vi "configure operation.vi"(7 "tag bus configurable plugin module configuration":refnum<class "Modbus Slave configuration.lvclass">, 8 "error in":errorcluster, 10 "line item in":T2, 11 "engine configuration":refnum<class "engine configuration.lvclass">) -> (0 "error out":errorcluster, 1 "success":bool, 2 "line item out":T2, 5 "changed":bool)   [LabVIEW 2013, in "Modbus Slave editor node.lvclass"]
doc: "Platypus Framework 1.0.1.65\nNI Systems Engineering - National Instruments"
uses:
  Modbus Slave editor node.lvclass
  permissions.ctl
  table line.ctl
  <vilib>/NI/TBM Modules/modbus slave/module channel/Modbus Module Channel.lvclass
  <vilib>/NI/Module Execution Interface/Engine Configuration/engine configuration.lvclass
  <vilib>/NI/TBM Modules/modbus slave/configuration/Modbus Slave configuration.lvclass
  <vilib>/NI/TBM Modules/modbus slave/module channel/data bank type.ctl
  <vilib>/NI/Tag Bus Module Framework/root configuration/TBM configuration.lvclass/TBM configuration.ctl
  <vilib>/NI/Tag Bus Module Framework/channel/TBM channel.lvclass/TBM channel.ctl
  <vilib>/NI/TBM Modules/modbus slave/module channel/Modbus Module Channel.lvclass/Modbus Module Channel.ctl
  <vilib>/NI/Tag Bus/tag/tag descriptor.lvclass/tag descriptor.ctl
  <vilib>/NI/Tag Bus/tag/Data Type.ctl
  <vilib>/NI/Tag Bus Module Framework/channel/Read channel classification.vi
  <vilib>/NI/TBM Modules/modbus slave/module channel/Read modbus type.vi
  <vilib>/NI/TBM Modules/modbus slave/module channel/Read starting address.vi
  <vilib>/NI/TBM Modules/modbus slave/module channel/Read subindex (bool).vi
  <vilib>/NI/Tag Bus/tag/read data type.vi
  <vilib>/NI/Tag Bus Module Framework/root configuration/Read instance name.vi
  <vilib>/NI/Tag Bus/tag/write data type.vi
  <vilib>/NI/Tag Bus Module Framework/channel/Write channel classification.vi
  <vilib>/NI/TBM Modules/modbus slave/module channel/Write modbus type.vi
  <vilib>/NI/TBM Modules/modbus slave/module channel/Write starting address.vi
  <vilib>/NI/TBM Modules/modbus slave/module channel/Write subindex (bool).vi
  <vilib>/NI/Tag Bus/tag/write tag name.vi
  <vilib>/NI/Tag Bus Module Framework/root configuration/create GUID.vi
  <vilib>/NI/Tag Bus/tag/tag descriptor.lvclass
panel:
  out "issues":string
  in  "Tag":i32(listbox)
  in  "Type":i32(listbox)
  in  "Bit":i32 min=0 max=15 step=1
  in  "Address (0 index)":i32
  in  "modbus bank":T1
  in  "cancel":bool
  in  "ok":bool
  in  "Access Type":T3
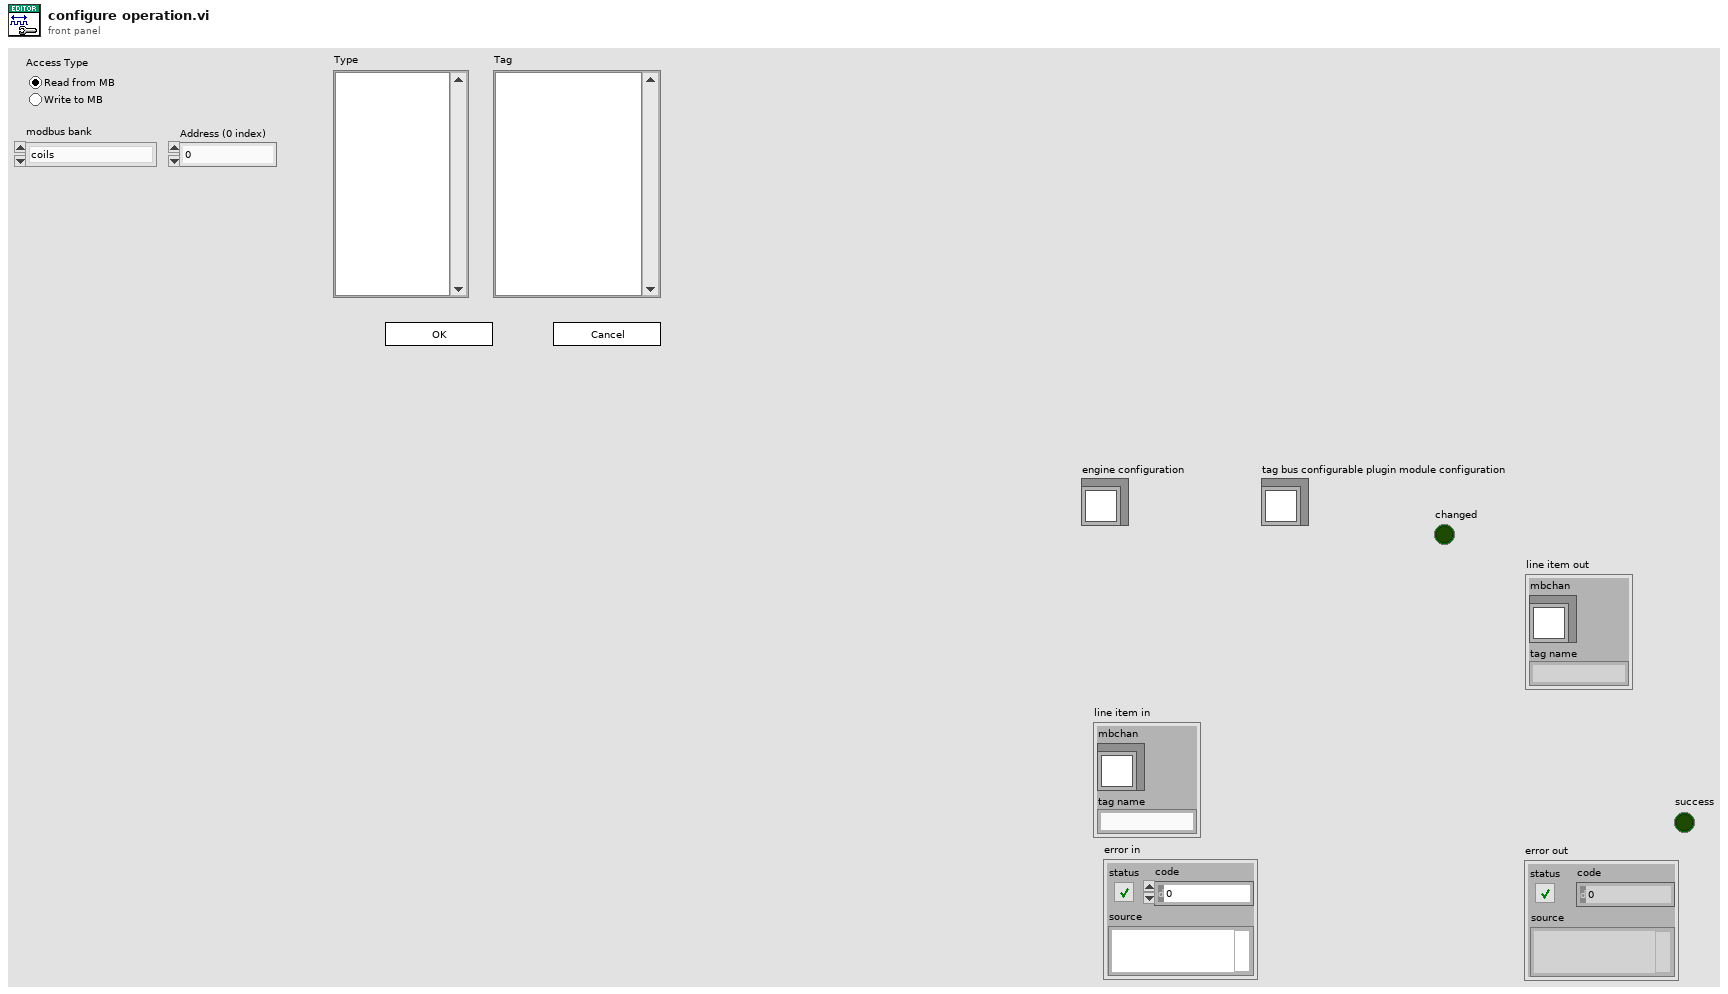
[diagram p1: front panel]
types:
  T1 = typedef "Modbus Module Channel.lvclass/data bank type.ctl" = enum16{"coils", "discrete inputs", "input registers", "holding registers"}
  T2 = typedef "Modbus Slave editor node.lvclass/table line.ctl" = cluster{"mbchan":refnum<class "Modbus Module Channel.lvclass">, "tag name":string}
  T3 = typedef "Modbus Slave editor node.lvclass/permissions.ctl" = enum32{"Read from MB", "Write to MB"}
  T4 = enum32{"Invalid", "Standard", "Closed", "Hidden", "Minimized", "Maximized"}
  T5 = enum32{"Invalid", "Default", "Floating", "Floating/Auto-Hide", "Modal"}
  T6 = enum8{"Enabled", "Disabled", "Disabled and Grayed Out"}
  T7 = typedef "tag bus.lvlib/tag descriptor.lvclass/Data Type.ctl" = enum16{"Double", "Single", "I64", "I32", "I16", "I8", "U64", "U32", "U16", "U8", "Boolean", "String", "Array of Double", "Array of Single", "Array of I64", "Array of I32", "Array of I16", "Array of I8", "Array of U64", "Array of U32", "Array of U16", "Array of U8", "Array of Boolean", "Array of String"}
  T8 = enum32{"invalid app kind", "Development System", "Run Time System", "Student Edition", "Embedded LabVIEW", "Evaluation", "Custom"}
  T9 = typedef "TBM channel.lvclass/channel classification.ctl" = enum16{"input data", "output data", "processing parameter", "processing result"}
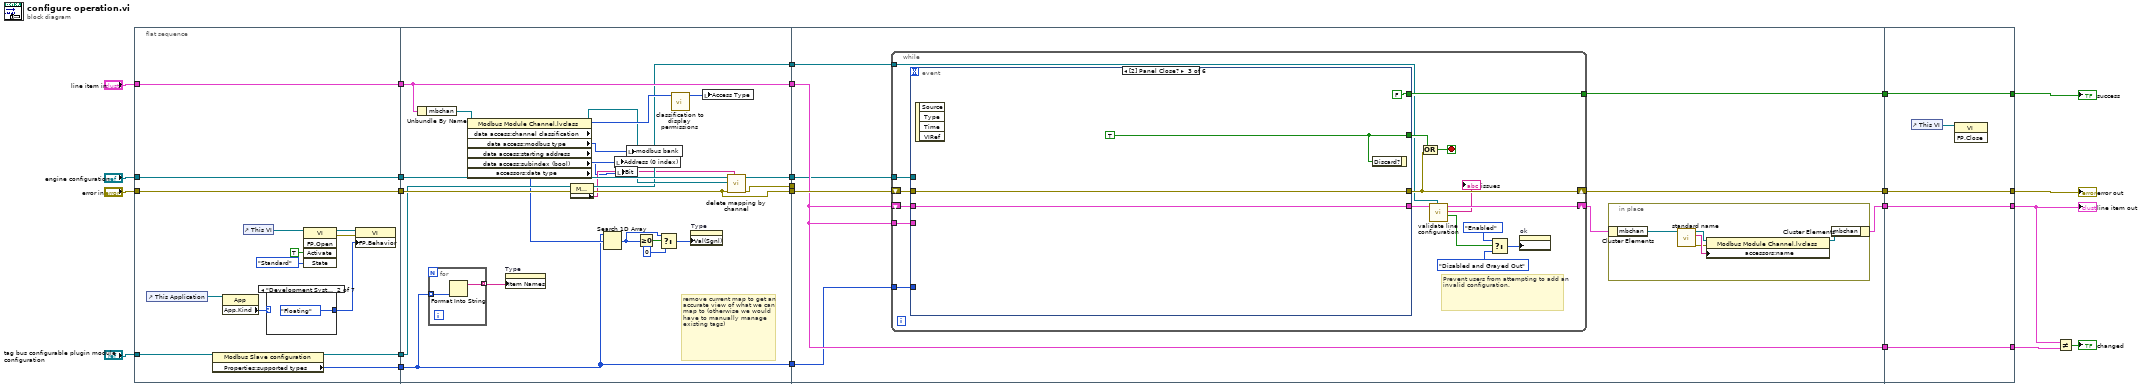
[diagram p0: block diagram]
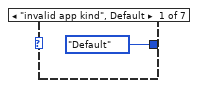
[diagram p2: hidden frame]
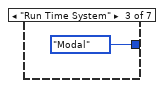
[diagram p3: hidden frame]
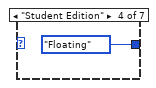
[diagram p4: hidden frame]
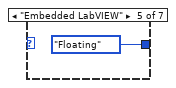
[diagram p5: hidden frame]
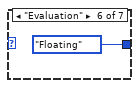
[diagram p6: hidden frame]
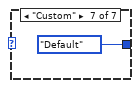
[diagram p7: hidden frame]
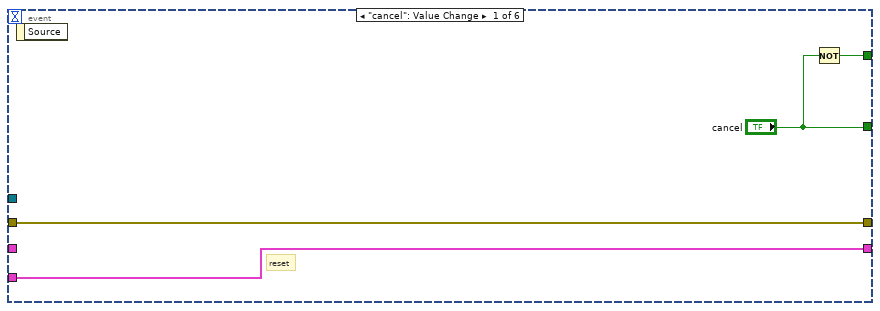
[diagram p8: hidden frame]
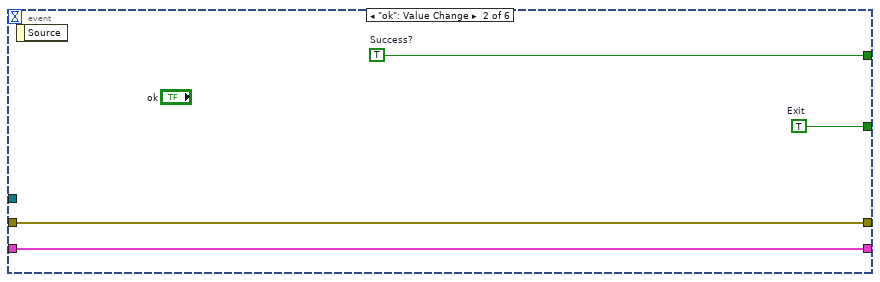
[diagram p9: hidden frame]
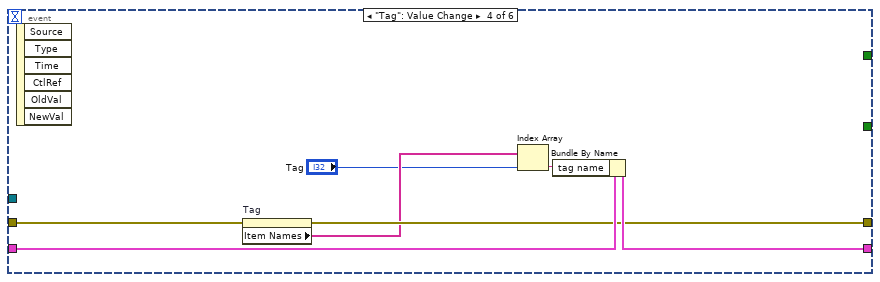
[diagram p10: hidden frame]
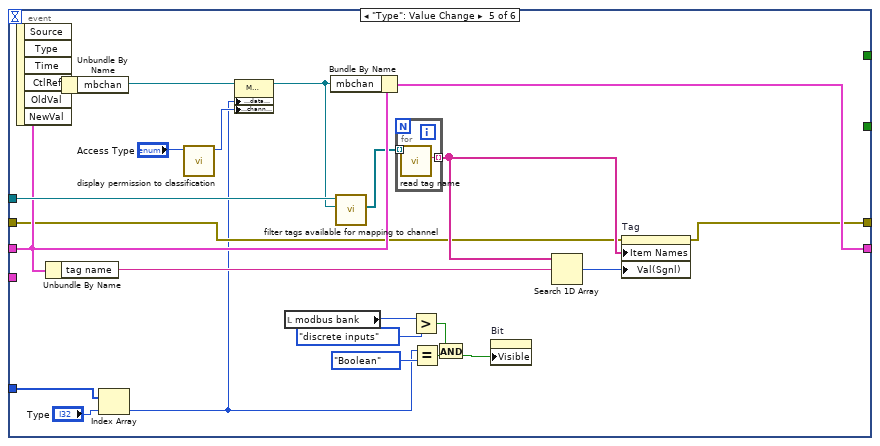
[diagram p11: hidden frame]
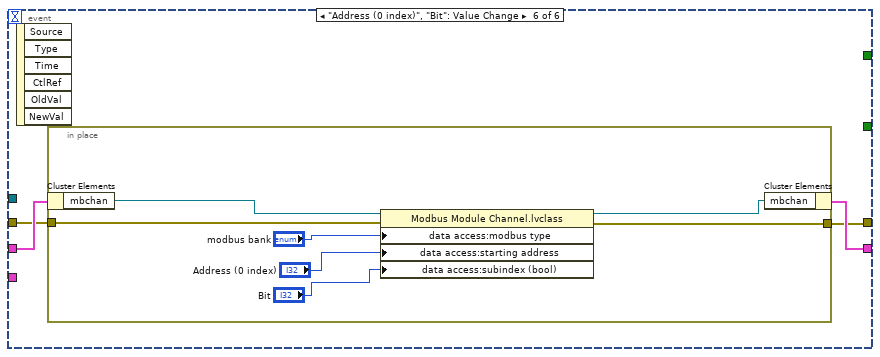
[diagram p12: hidden frame]
diagram:
  n1 = flat-sequence {
    tunnel: "line item in" -> [w37]
    tunnel: "error in" -> [w38]
    tunnel: [w38] -> w13
    tunnel: [w37] -> w12
    tunnel: [w28] -> w9
    tunnel: "engine configuration" -> [w28]
    tunnel: [w26] -> w6
    tunnel: "tag bus configurable plugin module configuration" -> [w27]
    tunnel: [w25] -> w2
    tunnel: w13 -> [w60]
    tunnel: w12 -> [w65]
    tunnel: [w65] -> w11
    tunnel: [w63] -> w10
    tunnel: w9 -> [w64]
    tunnel: [w57] -> w7
    tunnel: w6 -> [w58]
    tunnel: [w59] -> w4
    tunnel: [w61] -> w3
    tunnel: w2 -> [w47]
    tunnel: [w47] -> w1
    tunnel: [w78] -> w17
    tunnel: [w77] -> w16
    tunnel: [w72] -> w15
    tunnel: [w76] -> w14
    tunnel: w11 -> [w76]
    tunnel: w10 -> [w75]
    tunnel: w7 -> [w74]
    tunnel: w4 -> [w79]
    tunnel: w3 -> [_]
    tunnel: w1 -> [w71]
    tunnel: [w157] -> w18
    tunnel: [w158] -> w21
    tunnel: [w159] -> w22
    tunnel: [w160] -> w23
    tunnel: w17 -> [w160]
    tunnel: w16 -> [w159]
    tunnel: w15 -> [w158]
    tunnel: w14 -> [w157]
    frame #0 {
      n2 = control-ref of="This Application"() -> (w31:refnum<vi>)
      n3 = property class="Modbus Slave configuration"(reference=w27) -> (reference out=w26:refnum<class "Modbus Slave configuration.lvclass">, "Properties:supported types"=w25:T7[])  [unwired: 1 in, 1 out]
      n4 = property class="App"(reference=w31) -> ("App.Kind"=w30:T8)  [unwired: 1 in, 2 out]
      n5 = control-ref of="This VI"() -> (w32:refnum<vi>)
      n6 = case shown="\"Development System\"" w30 {
        tunnel: [T5."Default" ("Front Panel Window:Behavior") T5."Floating" ("Front Panel Window:Behavior") T5."Modal" ("Front Panel Window:Behavior") T5."Floating" ("Front Panel Window:Behavior") T5."Floating" ("Front Panel Window:Behavior") T5."Floating" ("Front Panel Window:Behavior") T5."Default" ("Front Panel Window:Behavior")] -> w29
        frame "invalid app kind", Default {
        }
        frame "Development System" {
        }
        frame "Run Time System" {
        }
        frame "Student Edition" {
        }
        frame "Embedded LabVIEW" {
        }
        frame "Evaluation" {
        }
        frame "Custom" {
        }
      }
      n7 = invoke class="VI" method="FP.Open"(reference=w32, "Activate"=TRUE ("Activate?"), "State"=T4."Standard") -> (reference out=w35:refnum<vi>, error out=w36:errorcluster)  [unwired: 2 in, 3 out]
      n8 = property class="VI"(reference=w35, error in=w36, "FP.Behavior"=w29) -> ()  [unwired: 2 out]
    }
    frame #1 {
      # "remove current map to get an accurate view of what we can map to (otherwise we would have to manually manage existing tags)"
      n9 = Unbundle By Name(w65) -> ("mbchan"=w67:refnum<class "Modbus Module Channel.lvclass">)
      n10 = for {
        tunnel: w47 -> [w70] mode=indexing
        tunnel: [w69] -> w46 mode=indexing
        n11 = Format Into String(w70) -> (resulting string=w69:string)  [unwired: 3 in, 1 out]
      }
      n12 = property class="Modbus Module Channel.lvclass"(reference=w67) -> (reference out=w62:refnum<class "Modbus Module Channel.lvclass">, "data access:channel classification"=w68:T9, "data access:modbus type"=w55:T1, "data access:starting address"=w54:u16, "data access:subindex (bool)"=w53:i32, "accessors:data type"=w52:T7)  [unwired: 1 in, 1 out]
      n13 = property on="Type" class="LstBox (strict)"("Item Names"=w46) -> ()  [unwired: 2 in, 2 out]
      n14 = property class="Modbus Slave configuration"(reference=w58, error in=w60) -> (reference out=w57:refnum<class "Modbus Slave configuration.lvclass">, error out=w59:errorcluster, "Properties:instance identifier"=w56:string)
      n15 = Search 1D Array(1D array=w47, element=w52) -> (index of element=w49:i32)  [unwired: 1 in]
      n16 = local write "Address (0 index)"(w54) -> ()
      n17 = local write "Bit"(w53) -> ()
      n18 = local write "modbus bank"(w55) -> ()
      n19 = Greater Or Equal To 0?(x=w49) -> (x >= 0?=w51:bool)
      n20 = Select(t=w49, s=w51, f=0) -> (s? t:f=w50:i32)
      n21 = call "classification to display permissions.vi"("channel classification"=w68) -> ("permissions"=w66:T3)  [unwired: 10 in]
      n22 = property on="Type" class="LstBox (strict)"("Val(Sgnl)"=w50) -> ()  [unwired: 2 in, 2 out]
      n23 = local write "Access Type"(w66) -> ()
      n24 = call <vilib>:"delete mapping by channel.vi"("owner ID"=w56, "error in"=w59, "channel"=w62, "engine configuration in"=w64) -> ("error out"=w61:errorcluster, "engine configuration out"=w63:refnum<class "engine configuration.lvclass">)  [unwired: 6 in]
    }
    frame #2 {
      n25 = while {
        shift-right: [w92] -> w77
        shift-left: w79 -> [w100]
        tunnel: [w99] -> w78
        shift-right: [w93] -> w73
        shift-left: w76 -> [w96]
        tunnel: w76 -> [w95]
        tunnel: w75 -> [w101]
        tunnel: w74 -> [w87]
        tunnel: w71 -> [w86]
        stop <- w97 stop-if-true
        # "Prevent users from attempting to add an invalid configuration."
        n26 = event shown="[2] Panel Close?" {
          selector: _ -> [_ _ _ _ _ _]
          dyn-events: _ -> [_ _ _ _ _ _]
          timeout: _ -> [_ _ _ _ _ _]
          tunnel: w101 -> [_ _ _ _ w139 _]
          tunnel: w100 -> [w105 w109 w113 w117 w125 w146]
          tunnel: [w105 w109 w113 w116 w124 w145] -> w92
          tunnel: [w104 w106 FALSE _ _ _] -> w99
          tunnel: ["cancel" w107 w111 _ _ _] -> w98
          tunnel: w96 -> [_ w108 w110 w120 w137 w148]
          tunnel: [w102 w108 w110 w119 w128 w147] -> w94
          tunnel: w95 -> [w102 _ _ _ _ _]
          tunnel: w86 -> [_ _ _ _ w122 _]
          event "cancel": Value Change {
            # "reset"
            n27 = event-data() -> ()  [unwired: 1 in, 1 out]
            n28 = Not(x="cancel") -> (.not. x?=w104:bool)
          }
          event "ok": Value Change {
            w106 = TRUE  # Success?
            w107 = TRUE  # Exit
            n29 = event-data() -> ()  [unwired: 1 in, 1 out]
          }
          event Panel Close? {
            w111 = TRUE ("cancel")
            n30 = event-data() -> ()  [unwired: 1 in, 4 out]
            n31 = event-data("Discard?"=w111) -> ()  [unwired: 1 in, 1 out]
          }
          event "Tag": Value Change {
            n32 = event-data() -> ()  [unwired: 1 in, 6 out]
            n33 = property on="Tag" class="LstBox (strict)"(error in=w117) -> (error out=w116:errorcluster, "Item Names"=w115:string[])  [unwired: 1 in, 1 out]
            n34 = Index Array(array=w115, index="Tag") -> (element=w118:string)
            n35 = Bundle By Name(cluster=w120, "tag name"=w118) -> (w119:T2)
          }
          event "Type": Value Change {
            n36 = event-data() -> ()  [unwired: 1 in, 6 out]
            n37 = Unbundle By Name(w137) -> ("tag name"=w129:string)
            n38 = Unbundle By Name(w137) -> ("mbchan"=w141:refnum<class "Modbus Module Channel.lvclass">)
            n39 = Index Array(array=w122, index="Type") -> (element=w121:T7)
            n40 = call "display permission to classification.vi"("display permissions"="Access Type") -> ("channel classification"=w140:T9)  [unwired: 10 in]
            n41 = property class="Modbus Module Channel.lvclass"(reference=w141, "accessors:data type"=w121, "data access:channel classification"=w140) -> (reference out=w138:refnum<class "Modbus Module Channel.lvclass">)  [unwired: 1 in, 1 out]
            n42 = local read "modbus bank"() -> (w133:T1)
            n43 = Bundle By Name(cluster=w137, "mbchan"=w138) -> (w128:T2)
            n44 = call <vilib>:"filter tags available for mapping to channel.vi"("channel to map to"=w138, "engine configuration in"=w139) -> ("filtered tags"=w136:refnum<class "tag descriptor.lvclass">[])  [unwired: 8 in, 1 out]
            n45 = for {
              tunnel: w136 -> [w144] mode=indexing
              tunnel: [w143] -> w126 mode=indexing
              n46 = call <vilib>:"read tag name.vi"("system tag in"=w144) -> ("name"=w143:string)  [unwired: 8 in, 2 out]
            }
            n47 = Greater?(x=w133, y=data_bank_type."discrete inputs") -> (0:w130:bool)
            n48 = Equal?(x=w121, y=Data_Type."Boolean") -> (x = y?=w134:bool)
            n49 = And(x=w130, y=w134) -> (x .and. y?=w131:bool)
            n50 = property on="Bit" class="DigNum (strict)"("Visible"=w131) -> ()  [unwired: 2 in, 2 out]
            n51 = Search 1D Array(1D array=w126, element=w129) -> (index of element=w127:i32)  [unwired: 1 in]
            n52 = property on="Tag" class="LstBox (strict)"(error in=w125, "Item Names"=w126, "Val(Sgnl)"=w127) -> (error out=w124:errorcluster)  [unwired: 1 in, 1 out]
          }
          event "Address (0 index)", "Bit": Value Change {
            n53 = event-data() -> ()  [unwired: 1 in, 6 out]
            n54 = in-place {
              in-place-border: w146 -> [w155]
              in-place-border: [w149] -> w145
              n55 = in-place-cluster #1(w148) -> ("mbchan"=w154:refnum<class "Modbus Module Channel.lvclass">)
              n56 = property class="Modbus Module Channel.lvclass"(reference=w154, error in=w155, "data access:modbus type"="modbus bank", "data access:starting address"="Address (0 index)", "data access:subindex (bool)"="Bit") -> (reference out=w150:refnum<class "Modbus Module Channel.lvclass">, error out=w149:errorcluster)
              n57 = in-place-cluster #1("mbchan"=w150) -> (w147:T2)
            }
          }
        }
        n58 = Compound Arithmetic op=OR(w98, w92) -> (w97:bool)
        n59 = call "validate line configuration.vi"("modbus"=w87, "line in"=w94) -> ("valid?"=w91:bool, "issues"=→"issues":string, "line out"=w93:T2)  [unwired: 7 in]
        n60 = Select(t=T6."Enabled" ("Disabled"), s=w91, f=T6."Disabled and Grayed Out") -> (s? t:f=w88:T6)
        n61 = property on="ok" class="Bool"("DisabledEnum"=w88) -> ()  [unwired: 2 in, 2 out]
      }
      n62 = in-place {
        n63 = in-place-cluster #2(w73) -> ("mbchan"=w81:refnum<class "Modbus Module Channel.lvclass">)
        n64 = call <vilib>:"standard name.vi"("Modbus Module Channel in"=w81) -> ("error out"=w83:errorcluster, "standard name"=w84:string, "Modbus Module Channel out"=w82:refnum<class "Modbus Module Channel.lvclass">)  [unwired: 8 in]
        n65 = property class="Modbus Module Channel.lvclass"(reference=w82, error in=w83, "accessors:name"=w84) -> (reference out=w80:refnum<class "Modbus Module Channel.lvclass">)  [unwired: 1 out]
        n66 = in-place-cluster #2("mbchan"=w80) -> (w72:T2)
      }
    }
    frame #3 {
      n67 = control-ref of="This VI"() -> (w156:refnum<vi>)
      n68 = invoke class="VI" method="FP.Close"(reference=w156) -> ()  [unwired: 2 in, 3 out]
    }
  }
  n69 = Not Equal?(x=w21, y=w18) -> (x != y?=→"changed":bool)
  "error out" <- w22
  "success" <- w23
  "line item out" <- w21
